vi "test Write and Read Float Array.vi"(8 "error in (no error)":errorcluster, 11 "TestCase in":refnum<class "Read Value Tests.lvclass">) -> (0 "error out":errorcluster, 3 "TestCase out":refnum<class "Read Value Tests.lvclass">)   [LabVIEW 2017, in "Pointer Tests.lvlib" / "Read Value Tests.lvclass"]
uses:
  Read Value Tests.lvclass
  Read Value Tests.lvclass/Read Value Tests.ctl
  Source/Classes/Pointer/Read 1D SGL.vi
  Source/Classes/Pointer/Read 1D DBL.vi
  <vilib>/addons/_JKI Toolkits/VI Tester/TestCase.llb/TestCase.lvclass
  Source/Classes/Pointer/Pointer.lvclass
  C:/Program Files (x86)/National Instruments/LabVIEW 2017/vi.lib/addons/_JKI Toolkits/VI Tester/TestCase.llb/TestCase.lvclass
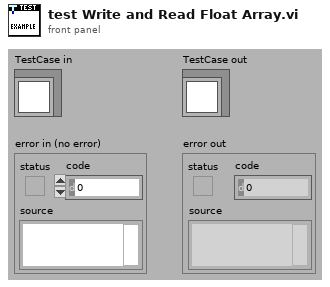
[diagram p1: front panel]
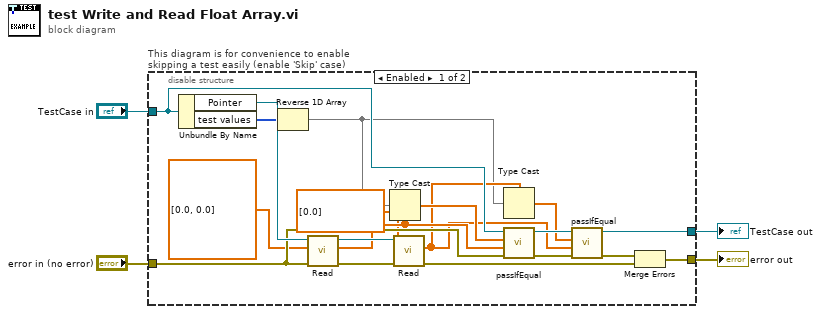
[diagram p0: block diagram]
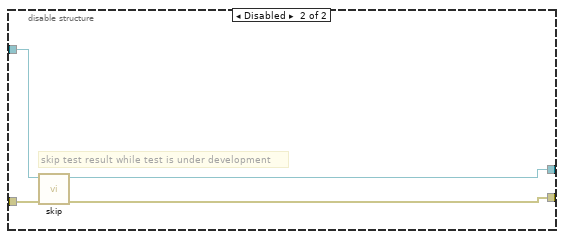
[diagram p2: hidden frame]
diagram:
  n1 = disable-structure "This diagram is for convenience to enable skipping a test easily (enable 'Skip' case)" shown="Enabled" {
    disable-tunnel: "TestCase in" -> [w15 w27]
    disable-tunnel: [w17 w25] -> w1
    disable-tunnel: [w12 w26] -> w3
    disable-tunnel: "error in (no error)" -> [w13 w24]
    frame Enabled {
      n2 = Unbundle By Name(w15) -> ("Pointer"=w14:refnum<class "Pointer.lvclass">, "test values"=w10:u8[])
      n3 = Reverse 1D Array(array=w10) -> (reversed array=w5:u8[])
      n4 = call-poly "Read.vi"("error in (no error)"=w13, "buffer in"=sgl[] [0.0, 0.0], "Pointer in"=w14) -> ("error out"=w18:errorcluster, "buffer out"=w9:sgl[], "Pointer out"=w20:refnum<class "Pointer.lvclass">)  [unwired: 5 in, 1 out]
      n5 = Type Cast(type=w9, x=w5) -> (*(type *) &x=w23:sgl[])
      n6 = call-poly "Read.vi"("error in (no error)"=w18, "buffer in"=dbl[] [0.0], "Pointer in"=w20) -> ("error out"=w11:errorcluster, "buffer out"=w8:dbl[])  [unwired: 5 in, 2 out]
      n7 = Type Cast(type=w8, x=w5) -> (*(type *) &x=w19:dbl[])
      n8 = call-dynamic "passIfEqual.vi"("error in (no error)"=w13, "y"=w9, "x"=w23, "TestCase in"=w15) -> ("error out"=w22:errorcluster, "TestCase out"=w21:refnum<class "Read Value Tests.lvclass">)  [unwired: 6 in]
      n9 = call-dynamic "passIfEqual.vi"("error in (no error)"=w22, "y"=w8, "x"=w19, "TestCase in"=w21) -> ("error out"=w16:errorcluster, "TestCase out"=w17:refnum<class "Read Value Tests.lvclass">)  [unwired: 6 in]
      n10 = Merge Errors(w16, w11) -> (w12:errorcluster)
    }
    frame Disabled {
      # "skip test result while test is under development"
      n11 = call <vilib>:"skip.vi"("error in (no error)"=w24, "TestCase in"=w27) -> ("error out"=w26:errorcluster, "TestCase out"=w25:refnum<class "Read Value Tests.lvclass">)  [unwired: 8 in]
    }
  }
  "error out" <- w3
  "TestCase out" <- w1
